vi "Tokenize JSON.vi"(11 "JSON String":string="{\n   \"data\":[\n      {\n         \"message\":{\n            \"content\":{\n               \"type\":\"text/plain\",\n               \"text\":\"Some text asd\"\n            },\n            \"subject\":\"My subject\",\n            \"status\":\"published\",\n            \"replyCount\":4.8,\n            \"likeCount\":0.7\n         }\n      }\n   ]\n}") -> (2 "Variable Names":string[](array[string]), 3 "Token Array":T1[](array[typedef]))   [LabVIEW 2026]
uses:
  Token.ctl
  <vilib>/regexp/Match Regular Expression.xnode
panel:
  out "Array":string[](array[string])
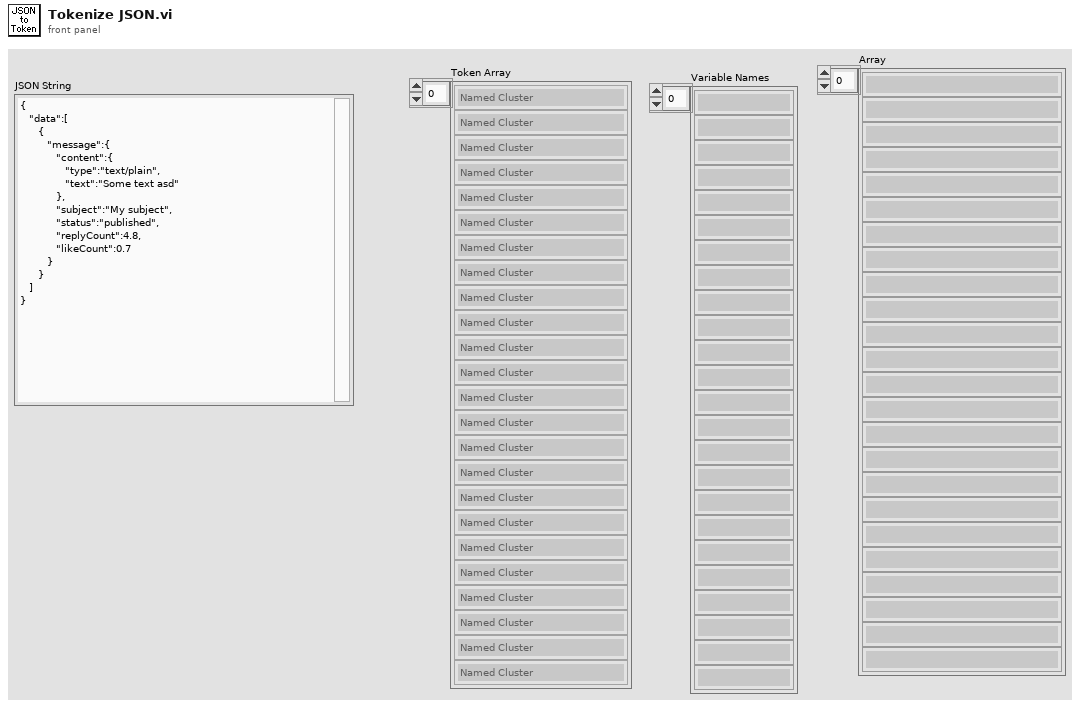
[diagram p1: front panel]
types:
  T1 = typedef "Token.ctl" = enum16{"End", "Boolean", "Named Cluster", "Unnamed Cluster", "Array", "String", "Decimal", "FloatingPoint", "End Array", "End Cluster"}
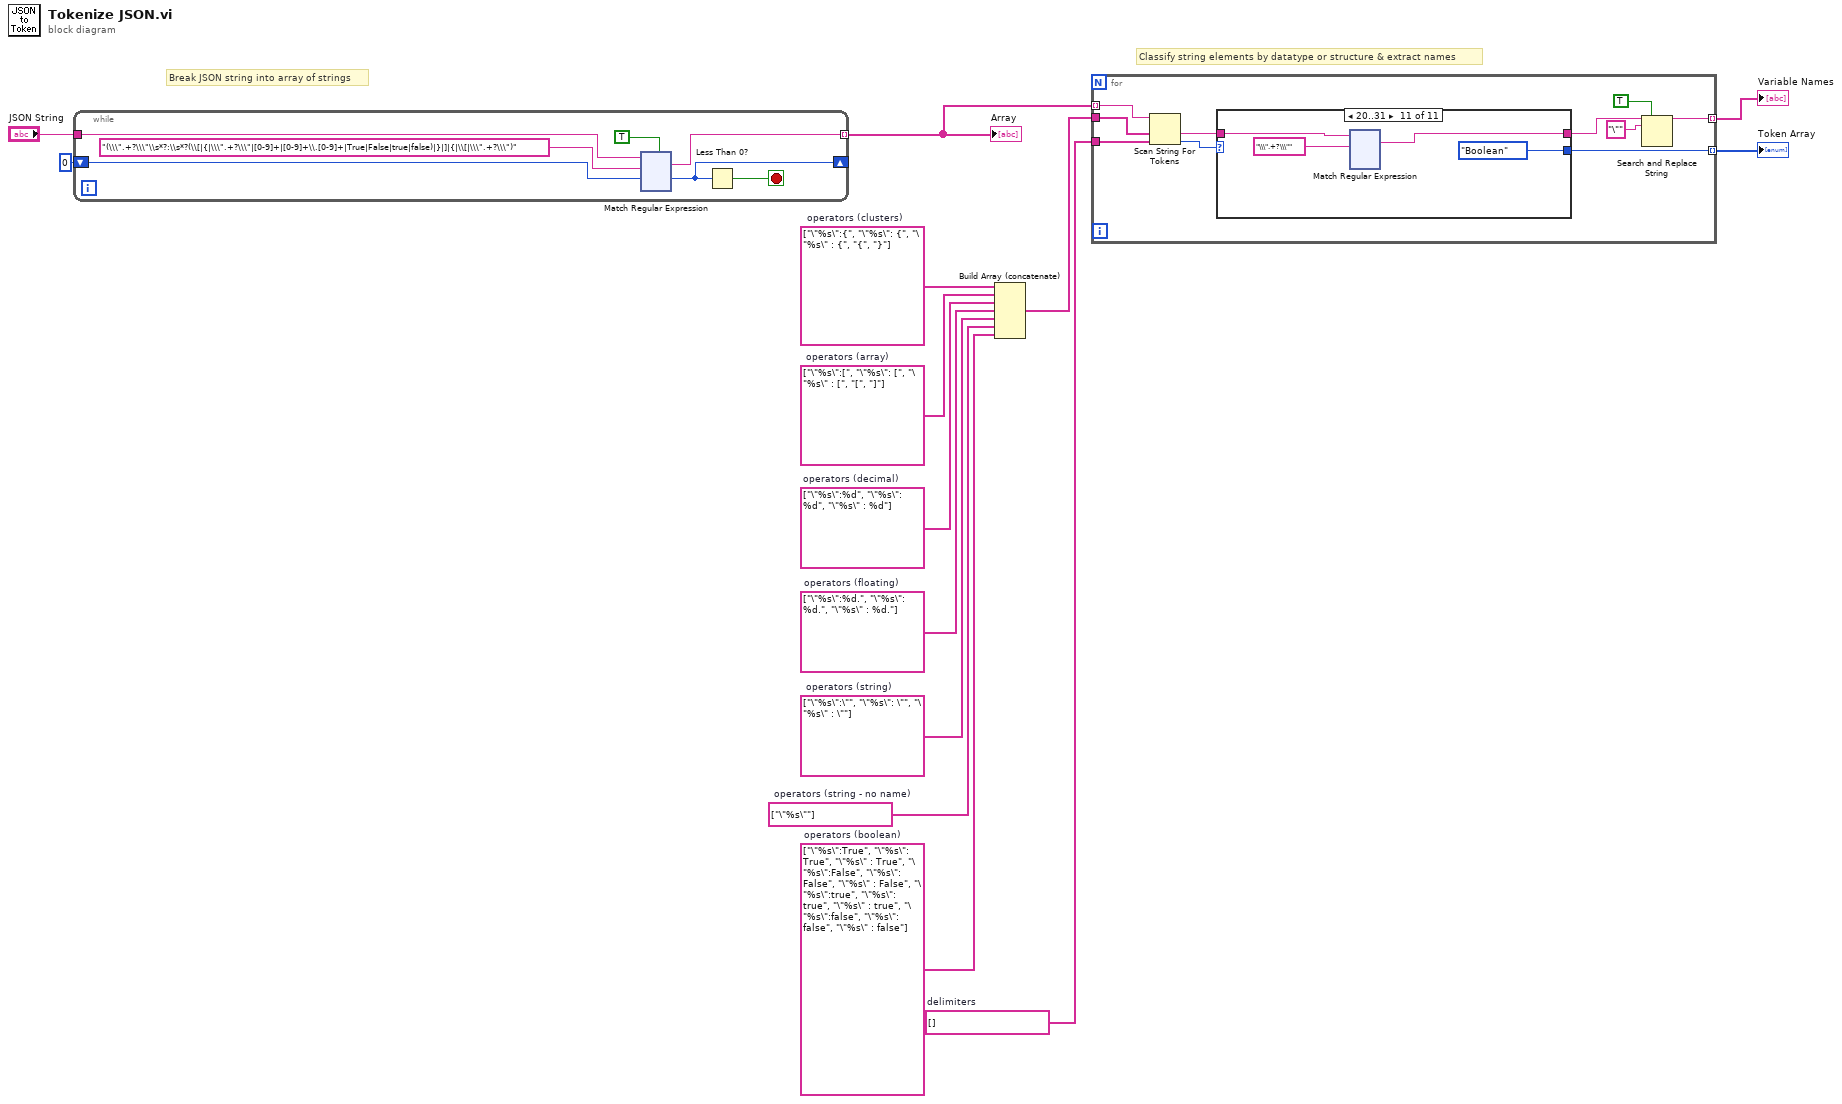
[diagram p0: block diagram]
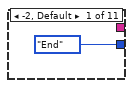
[diagram p2: hidden frame]
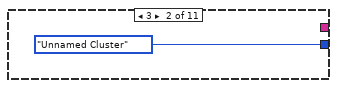
[diagram p3: hidden frame]
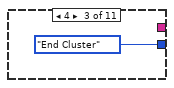
[diagram p4: hidden frame]
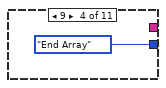
[diagram p5: hidden frame]
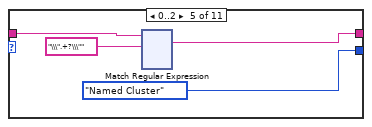
[diagram p6: hidden frame]
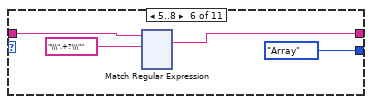
[diagram p7: hidden frame]
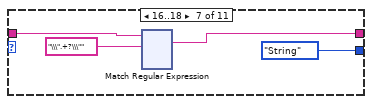
[diagram p8: hidden frame]
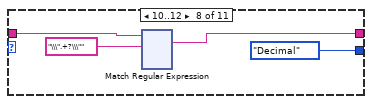
[diagram p9: hidden frame]
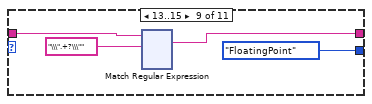
[diagram p10: hidden frame]
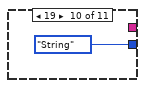
[diagram p11: hidden frame]
diagram:
  w1 = string[] ["\"%s\":True", "\"%s\": True", "\"%s\" : True", "\"%s\":False", "\"%s\": False", "\"%s\" : False", "\"%s\":true", "\"%s\": true", "\"%s\" : true", "\"%s\":false", "\"%s\": false", "\"%s\" : false"]  # operators (boolean)
  w3 = string[] ["\"%s\""]  # operators (string - no name)
  w4 = string[] ["\"%s\":\"", "\"%s\": \"", "\"%s\" : \""]  # operators (string)
  w5 = string[] ["\"%s\":%d.", "\"%s\": %d.", "\"%s\" : %d."]  # operators (floating)
  w6 = string[] ["\"%s\":%d", "\"%s\": %d", "\"%s\" : %d"]  # operators (decimal)
  w7 = string[] ["\"%s\":[", "\"%s\": [", "\"%s\" : [", "[", "]"]  # operators (array)
  w8 = string[] ["\"%s\":{", "\"%s\": {", "\"%s\" : {", "{", "}"]  # operators (clusters)
  w12 = string[] []  # delimiters
  # "Classify string elements by datatype or structure & extract names"
  # "Break JSON string into array of strings"
  n1 = while {
    tunnel: "JSON String" -> [w20]
    shift-right: [w15] -> _
    shift-left: 0 ("offset past match") -> [w18]
    tunnel: [w17] -> w11 mode=indexing
    stop <- w21 stop-if-true
    n2 = xnode "Match Regular Expression"("input string"=w20, "regular expression"="(\\\".+?\\\"\\s*?:\\s*?(\\[|{|\\\".+?\\\"|[0-9]+|[0-9]+\\.[0-9]+|True|False|true|false)|}|]|{|\\[|\\\".+?\\\")", "offset (0)"=w18, "multiline? (F)"=TRUE) -> ("whole match"=w17:string, "offset past match"=w15:i32)  [unwired: 2 in, 3 out]
    n3 = Less Than 0?(x=w15) -> (x < 0?=w21:bool)
  }
  "Array" <- w11
  n4 = Build Array (concatenate)(w8, w7, w6, w5, w4, w3, w1) -> (w2:string[])
  n5 = for {
    tunnel: w11 -> [w148] mode=indexing
    tunnel: w12 -> [w147]
    tunnel: w2 -> [w146]
    tunnel: [w144] -> w10 mode=indexing
    tunnel: [w141] -> w9 mode=indexing
    n6 = Scan String For Tokens(6:w147, 7:w146, 9:w148) -> (0:w145:i32, 1:w143:string)  [unwired: 3 in, 2 out]
    n7 = case shown="20..31" w145 {
      tunnel: [Token."End" Token."Unnamed Cluster" Token."End Cluster" Token."End Array" Token."Named Cluster" Token."Array" Token."String" Token."Decimal" Token."FloatingPoint" Token."String" Token."Boolean"] -> w144
      tunnel: w143 -> [_ _ _ _ w154 w275 w396 w517 w638 _ w760]
      tunnel: [_ _ _ _ w153 w274 w395 w516 w637 _ w759] -> w142
      frame -2, Default {
      }
      frame 3 {
      }
      frame 4 {
      }
      frame 9 {
      }
      frame 0..2 {
        n8 = xnode "Match Regular Expression"("input string"=w154, "regular expression"="\\\".+?\\\"") -> ("whole match"=w153:string)  [unwired: 4 in, 4 out]
      }
      frame 5..8 {
        n9 = xnode "Match Regular Expression"("input string"=w275, "regular expression"="\\\".+?\\\"") -> ("whole match"=w274:string)  [unwired: 4 in, 4 out]
      }
      frame 16..18 {
        n10 = xnode "Match Regular Expression"("input string"=w396, "regular expression"="\\\".+?\\\"") -> ("whole match"=w395:string)  [unwired: 4 in, 4 out]
      }
      frame 10..12 {
        n11 = xnode "Match Regular Expression"("input string"=w517, "regular expression"="\\\".+?\\\"") -> ("whole match"=w516:string)  [unwired: 4 in, 4 out]
      }
      frame 13..15 {
        n12 = xnode "Match Regular Expression"("input string"=w638, "regular expression"="\\\".+?\\\"") -> ("whole match"=w637:string)  [unwired: 4 in, 4 out]
      }
      frame 19 {
      }
      frame 20..31 {
        n13 = xnode "Match Regular Expression"("input string"=w760, "regular expression"="\\\".+?\\\"") -> ("whole match"=w759:string)  [unwired: 4 in, 4 out]
      }
    }
    n14 = Search and Replace String(replace all?=TRUE ("replace all? (F)"), input string=w142, search string="\"") -> (result string=w141:string)  [unwired: 5 in, 3 out]
  }
  "Token Array" <- w10
  "Variable Names" <- w9
